vi "CmdExe.Launch Executable with Timeout, Abort, and Error Checks - Using DotNet Process.vi"(5 "Cmd IN Ref":refnum<vi>, 6 "Setup":T1={"Timeout (s)"=60.0, "Show Cmd Win"=FALSE, "Error Check"={"StdOut_Ck"=FALSE, "StdOutErrMsgs"=["Error", "Unable to find device "], "StdErr_Ck"=FALSE, "RtnCode_Ck"=FALSE, "RtnCodePASS"=0}, "Log_En"=FALSE, "LogFileName"="", "LogDir"=path ""}, 7 "Output Ref":refnum<vi>, 8 "error in (no error)":errorcluster, 9 "Ignore StdErr":bool, 10 "Args":string="/InputFile JSONFILE /SerialDevice /OutputDevice /NoBackup", 11 "Executable":path=path "C:/MTE/FW Load and Display Cal/Config/Bin/utahev_0_7/lighthouse_configtool.exe") -> (0 "error out":errorcluster, 1 "Duration(s)":dbl, 3 "Data Out":string)   [LabVIEW 2018]
uses:
  <vilib>/KATE/Time/Time Utils.lvlib
  Errors/Error.Error Code List.ctl
  <vilib>/KATE/Files/File Utils.lvlib
  CmdConsole/CmdConsole.lvclass
  CmdExe.Setup Params.ctl
  CmdExe.Output Error Check Setup.ctl
panel:
  out "return code":i32
  out "Cmd":string
  out "Done":bool
  # "Launch Exe"
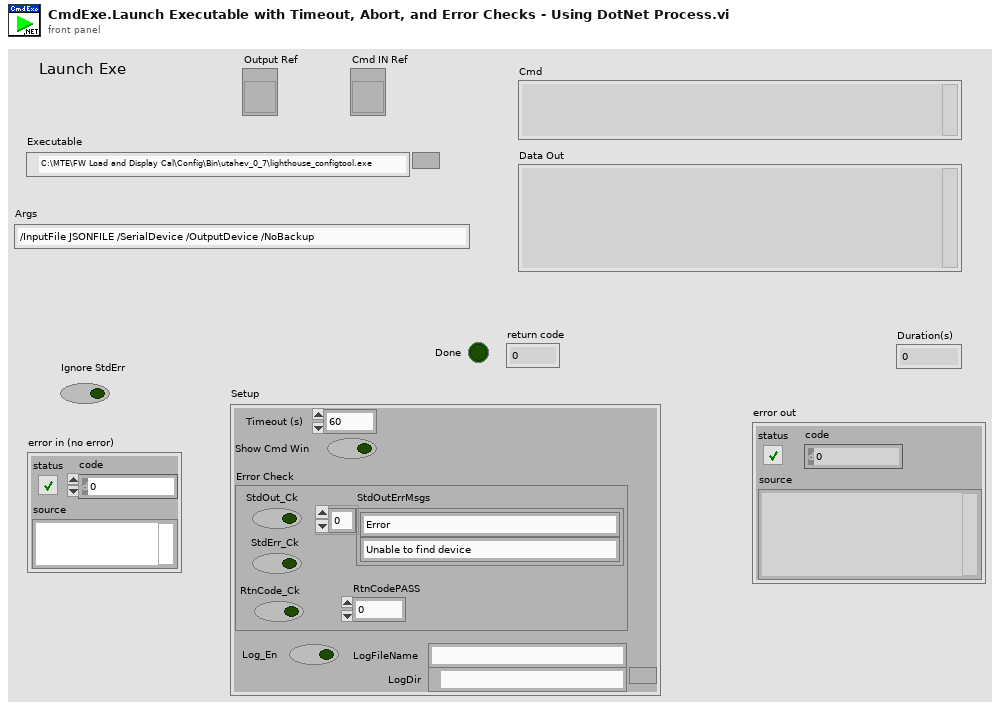
[diagram p1: front panel]
types:
  T1 = typedef "CmdExe.Setup Params.ctl" = cluster{"Timeout (s)":dbl, "Show Cmd Win":bool, "Error Check":T2, "Log_En":bool, "LogFileName":string, "LogDir":path}
  T2 = typedef "CmdExe.Output Error Check Setup.ctl" = cluster{"StdOut_Ck":bool, "StdOutErrMsgs":string[], "StdErr_Ck":bool, "RtnCode_Ck":bool, "RtnCodePASS":i32}
  T3 = enum16{"open", "replace", "create", "open or create", "replace or create", "replace or create with confirmation"}
  T4 = cluster{"Exe":string, "StdOut":string, "StdError":string, "LogFile":path, "Args":string, "TimedOut":bool, "RtnCode":i32, "LogEn":bool}
  T5 = typedef "Error.Error Code List.ctl" = i32
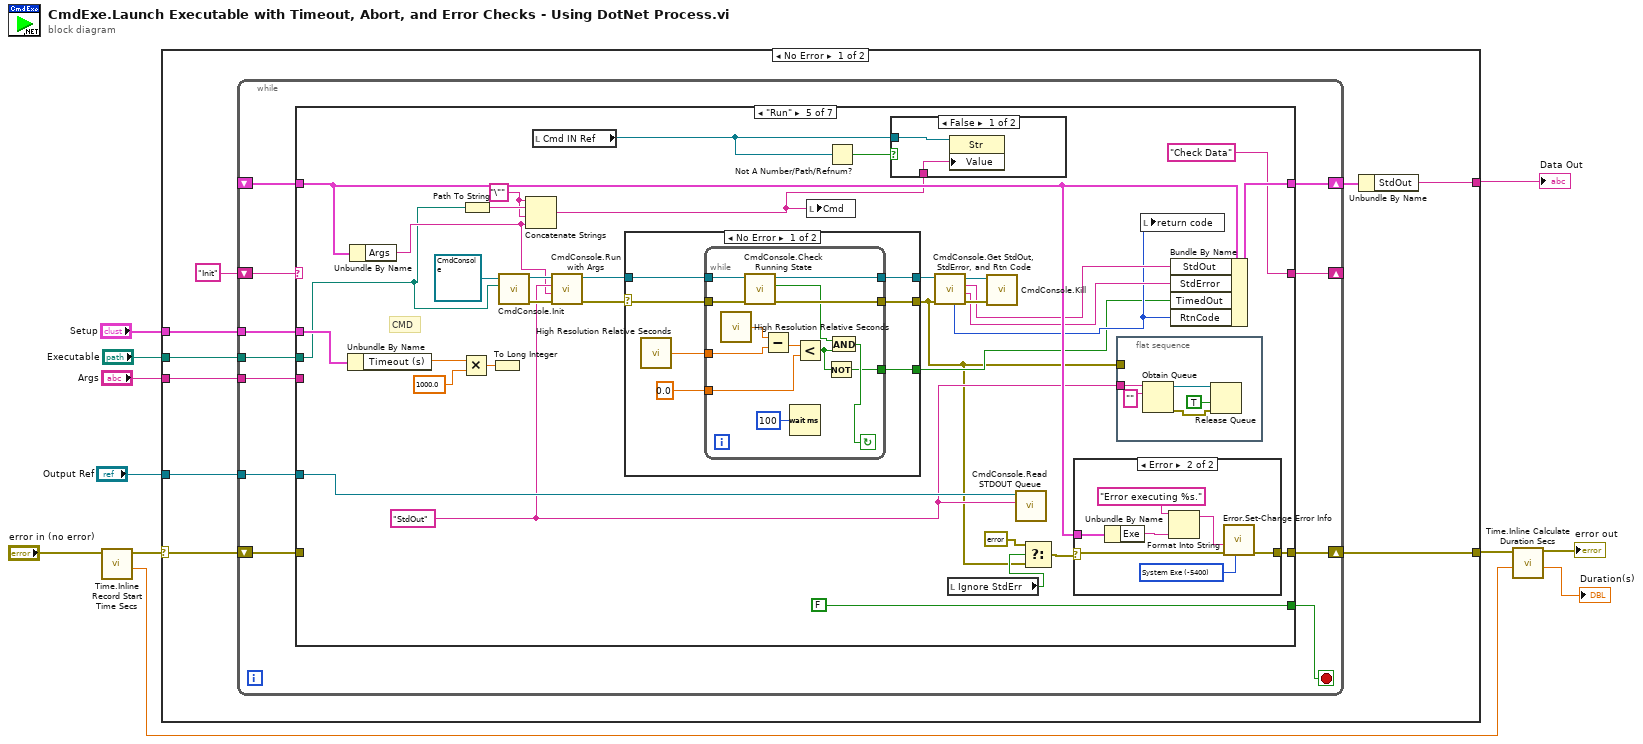
[diagram p0: block diagram]
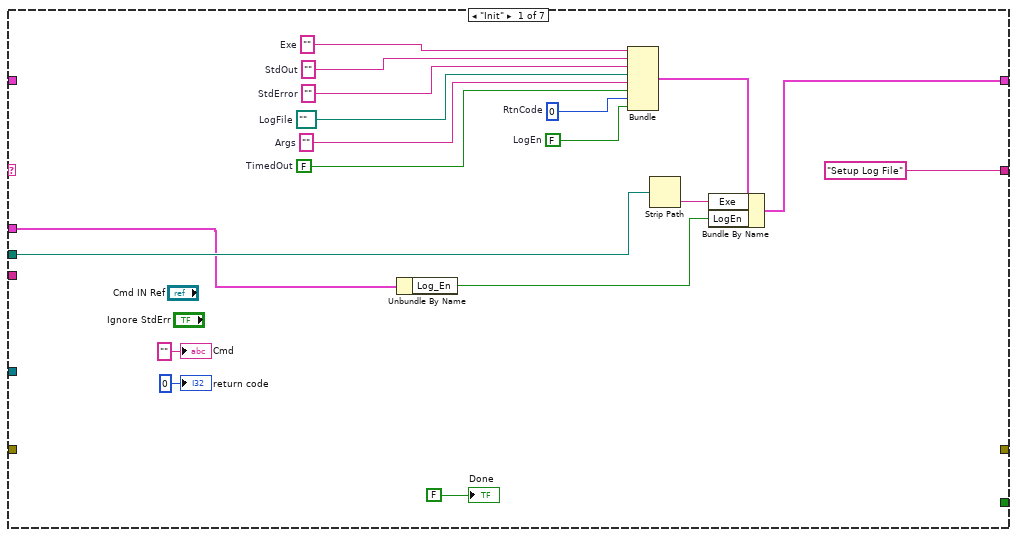
[diagram p2: hidden frame]
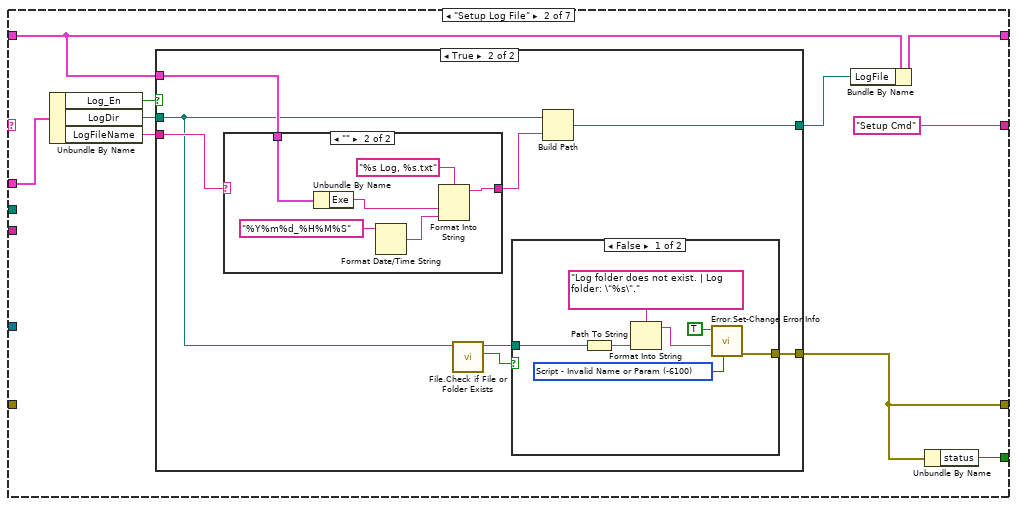
[diagram p3: hidden frame]
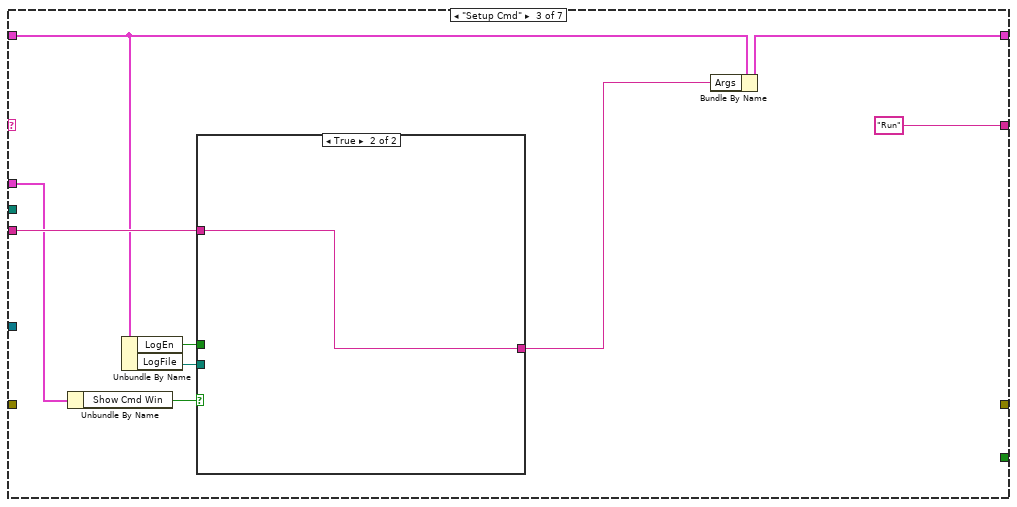
[diagram p7: hidden frame]
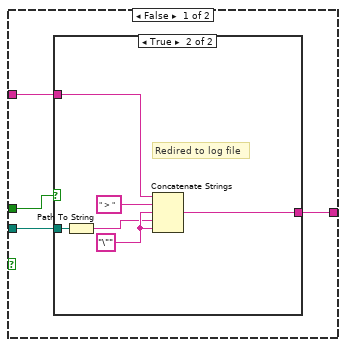
[diagram p8: hidden frame]
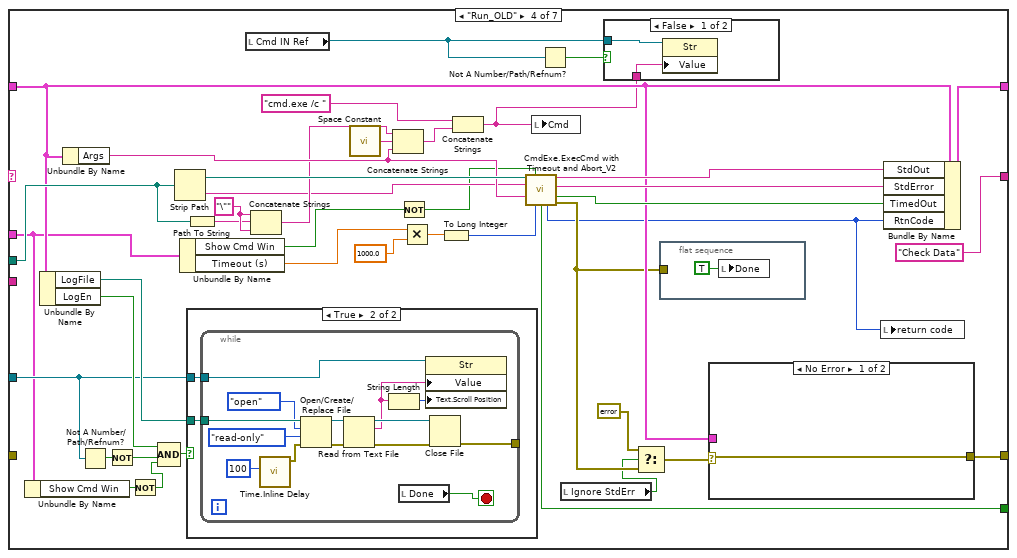
[diagram p10: hidden frame]
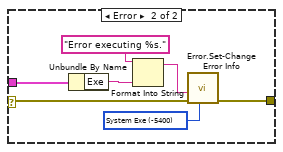
[diagram p11: hidden frame]
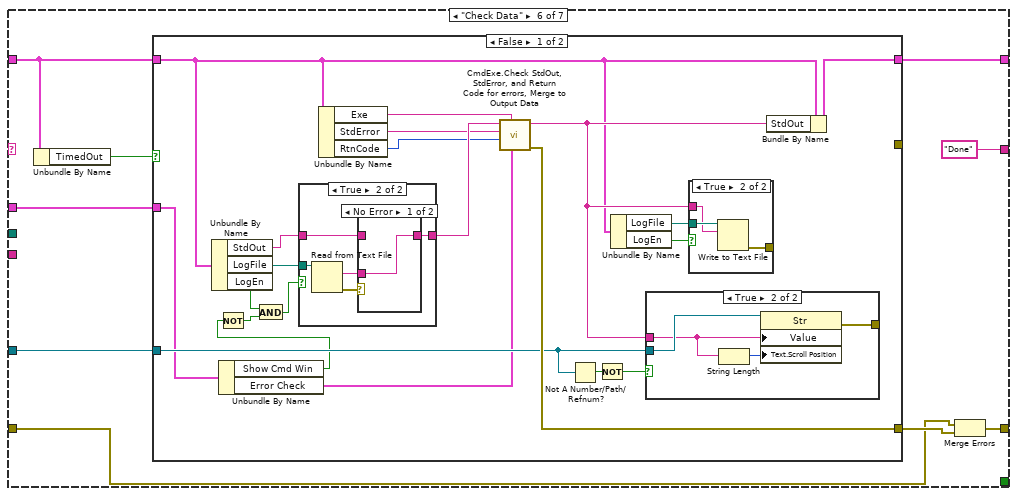
[diagram p17: hidden frame]
diagram:
  n1 = call <vilib>:"Time.Inline Record Start Time Secs.vi"("Error In Upper"="error in (no error)") -> ("Start(s)"=w8:dbl, "Error Out Upper"=w11:errorcluster)  [unwired: 8 in, 1 out]
  n2 = case shown="No Error" w11 {
    selector: w11 -> [w19 w318]
    tunnel: [w18 w318] -> w10
    tunnel: [w16 _] -> w9
    tunnel: "Executable" -> [w15 _]
    tunnel: "Args" -> [w14 _]
    tunnel: "Setup" -> [w13 _]
    tunnel: "Output Ref" -> [w12 _]
    frame No Error {
      n3 = while {
        shift-right: [w29] -> w17
        shift-left: _ -> [w28]
        shift-right: [w21] -> _
        shift-left: "Init" -> [w31]
        shift-right: [w27] -> w18
        shift-left: w19 -> [w30]
        tunnel: w15 -> [w25]
        tunnel: w14 -> [w24]
        tunnel: w13 -> [w23]
        tunnel: w12 -> [w22]
        stop <- w26 stop-if-true
        n4 = case shown="\"Run\"" w31 {
          tunnel: ["Setup Log File" "Setup Cmd" "Run" "Check Data" "Check Data" "Done" "Done"] -> w21
          tunnel: w30 -> [_ _ _ _ _ w242 w314]
          tunnel: [w38 w58 w89 w143 w204 w250 w315] -> w29
          tunnel: [_ w51 _ w114 w196 w244 w314] -> w27
          tunnel: w28 -> [_ w56 w84 w113 w195 w248 w315]
          tunnel: [_ w50 _ w139 FALSE _ TRUE] -> w26
          tunnel: w25 -> [w41 _ _ w127 w177 _ _]
          tunnel: w24 -> [_ _ w87 _ _ _ _]
          tunnel: w23 -> [w35 w55 w83 w109 w192 w246 _]
          tunnel: w22 -> [_ _ _ w115 w197 w249 _]
          frame "Init" {
            w36 = FALSE  # LogEn
            w37 = 0  # RtnCode
            w42 = FALSE  # TimedOut
            w43 = ""  # Args
            w44 = path ""  # LogFile
            w45 = ""  # StdError
            w46 = ""  # StdOut
            w48 = ""  # Exe
            n5 = Unbundle By Name(w35) -> ("Log_En"=w34:bool)
            n6 = Bundle("Exe"=w48, "StdOut"=w46, "StdError"=w45, "LogFile"=w44, "Args"=w43, "TimedOut"=w42, "RtnCode"=w37, "LogEn"=w36) -> (w39:T4)  [unwired: 1 in]
            n7 = Strip Path(path=w41) -> (name=w40:string)  [unwired: 1 out]
            n8 = Bundle By Name(cluster=w39, "Exe"=w40, "LogEn"=w34) -> (w38:T4)
            "Done" <- FALSE ("Done")
            "Cmd" <- "" ("Cmd")
            "return code" <- 0 ("return code")
          }
          frame "Setup Log File" {
            n9 = Unbundle By Name(w55) -> ("Log_En"=w54:bool, "LogDir"=w53:path, "LogFileName"=w52:string)
            n10 = case shown="True" w54 {
              tunnel: [_ w67] -> w57
              tunnel: w56 -> [_ w65]
              tunnel: w53 -> [_ w61]
              tunnel: w52 -> [_ w64]
              tunnel: [_ w60] -> w51
              frame False {
              }
              frame True {
                n11 = case shown="\"\"" w64 {
                  selector: w64 -> [w75 _]
                  tunnel: [w75 w78] -> w66
                  tunnel: w65 -> [_ w77]
                  frame Default {
                  }
                  frame "" {
                    n12 = Unbundle By Name(w77) -> ("Exe"=w76:string)
                    n13 = Format Date/Time String(time format string (%c)="%Y%m%d_%H%M%S") -> (date/time string=w81:string)  [unwired: 2 in]
                    n14 = Format Into String(format string="%s Log, %s.txt", w76, w81) -> (resulting string=w78:string)  [unwired: 2 in, 1 out]
                  }
                }
                n15 = call <vilib>:"File.Check if File or Folder Exists.vi"("Path"=w61) -> ("Exists"=w62:bool, "Dup Path"=w63:path)  [unwired: 6 in, 3 out]
                n16 = case shown="False" w62 {
                  tunnel: [w68 _] -> w60
                  tunnel: w63 -> [w72 _]
                  frame False {
                    w70 = T5 -6100 items=["No Error"=0, "Abort"=-2, "Misc"=-5000, "Fixture Error"=-5100, "File IO - General"=-5200, "FIle IO - Config Error"=-5201, "Instrument - General"=-5300, "Instrument - Serial Com"=-5301, "Instrument - Camera"=-5302, "Instrument - PS"=-5303, "Instrument - Oscilloscope"=-5304, "Instrument - Function Gen"=-5305, "Instrument - Load"=-5306, "Instrument - Meter"=-5307, "Instrument - Power Control"=-5308, "Instrument - Motion"=-5309, "Instrument - RF"=-5310, "System Exe"=-5400, "Image Processing"=-5500, "Communication"=-5600, "Script - Syntax Error"=-6000, "Script - Invalid Name or Param"=-6100, "Script - Timeout"=-6200, "Invalid Data"=-6300] ("Std Code")
                    n17 = Path To String(path=w72) -> (string=w73:string)
                    n18 = Format Into String(format string="Log folder does not exist. | Log folder: \"%s\".", w73) -> (resulting string=w69:string)  [unwired: 2 in, 1 out]
                    n19 = call "Error.Set-Change Error Info.vi"("Std Code"=w70, "Description"=w69, "Set Error"=TRUE) -> ("error out"=w68:errorcluster)  [unwired: 8 in]
                  }
                  frame True {
                    # "Folders exist.\nNo error."
                  }
                }
                n20 = Build Path(base path=w61, name or relative path=w66) -> (appended path=w67:path)
              }
            }
            n21 = Bundle By Name(cluster=w56, "LogFile"=w57) -> (w58:T4)
            n22 = Unbundle By Name(w51) -> ("status"=w50:bool)
          }
          frame "Setup Cmd" {
            n23 = Unbundle By Name(w83) -> ("Show Cmd Win"=w82:bool)
            n24 = Unbundle By Name(w84) -> ("LogEn"=w85:bool, "LogFile"=w88:path)
            n25 = case shown="True" w82 {
              tunnel: w88 -> [w94 _]
              tunnel: w87 -> [w93 w102]
              tunnel: [w92 w102] -> w86
              tunnel: w85 -> [w91 _]
              frame False {
                n26 = case shown="True" w91 {
                  tunnel: w94 -> [_ w98]
                  tunnel: w93 -> [w95 w97]
                  tunnel: [w95 w96] -> w92
                  frame False {
                  }
                  frame True {
                    w101 = "\""
                    # "Redired to log file"
                    n27 = Path To String(path=w98) -> (string=w100:string)
                    n28 = Concatenate Strings(w97, " > ", w101, w100, w101) -> (w96:string)
                  }
                }
              }
              frame True {
              }
            }
            n29 = Bundle By Name(cluster=w84, "Args"=w86) -> (w89:T4)
          }
          frame "Run_OLD" {
            w128 = "\""
            n30 = Unbundle By Name(w109) -> ("Show Cmd Win"=w108:bool)
            n31 = Unbundle By Name(w113) -> ("LogFile"=w134:path, "LogEn"=w120:bool)
            n32 = Unbundle By Name(w113) -> ("Args"=w129:string)
            n33 = Not A Number/Path/Refnum?(number/path/refnum=w115) -> (NaN/Path/Refnum?=w123:bool)
            n34 = Not(x=w123) -> (.not. x?=w122:bool)
            n35 = Not(x=w108) -> (.not. x?=w107:bool)
            n36 = Compound Arithmetic op=AND(w120, w122, w107) -> (w121:bool)
            n37 = Strip Path(path=w127) -> (stripped path=w133:path, name=w124:string)
            n38 = Unbundle By Name(w109) -> ("Show Cmd Win"=w118:bool, "Timeout (s)"=w119:dbl)
            n39 = Path To String(path=w127) -> (string=w126:string)
            n40 = case shown="True" w121 {
              tunnel: w134 -> [_ w155]
              tunnel: w115 -> [_ w156]
              frame False {
              }
              frame True {
                n41 = while {
                  tunnel: w156 -> [w162]
                  tunnel: w155 -> [w166]
                  tunnel: [w165] -> _
                  stop <- w161 stop-if-true
                  n42 = call <vilib>:"Time.Inline Delay.vi"("Wait(ms)"=u32 100) -> ("error out top"=w159:errorcluster)  [unwired: 9 in, 1 out]
                  n43 = Open/Create/Replace File(file path (use dialog)=w166, error in=w159, operation (0:open)=T3."open", access (0:read/write)=enum16{"read/write", "read-only", "write-only"}."read-only") -> (refnum out=w167:refnum<file>, error out=w170:errorcluster)  [unwired: 2 in, 1 out]
                  n44 = Read from Text File(file (use dialog)=w167, error in=w170) -> (refnum out=w168:refnum<file>, text=w158:string, error out=w169:errorcluster)  [unwired: 2 in, 1 out]
                  n45 = String Length(string=w158) -> (length=w157:i32)
                  n46 = local read "Done"() -> (w161:bool)
                  n47 = property class="Str"(reference=w162, "Value"=w158, "Text.Scroll Position"=w157) -> ()  [unwired: 1 in, 2 out]
                  n48 = Close File(refnum=w168, error in=w169) -> (error out=w165:errorcluster)  [unwired: 1 out]
                }
              }
            }
            n49 = local read "Cmd IN Ref"() -> (w106:refnum<vi>)
            n50 = Concatenate Strings(w128, w126, w128) -> (w125:string)
            n51 = call <vilib>:"Space Constant.vi"() -> ("String"=w130:string)
            n52 = Concatenate Strings(w125, w130, w129) -> (w131:string)
            n53 = Not(x=w118) -> (.not. x?=w117:bool)
            n54 = Multiply(x=w119, y=1000.0) -> (x*y=w138:dbl)
            n55 = To Long Integer(number=w138) -> (32bit integer=w136:i32)
            n56 = Concatenate Strings("cmd.exe /c ", w131) -> (w103:string)
            n57 = call "CmdExe.ExecCmd with Timeout and Abort_V2.vi"("Working Dir"=w133, "Run minimized? (T)"=w117, "Executable"=w124, "Arguements"=w129, "Timeout ms(-1)"=w136) -> ("STD OUT"=w116:string, "STD ERR"=w142:string, "Timed Out"=w141:bool, "Aborted"=w139:bool, "return code"=w104:i32, "error out"=w112:errorcluster)  [unwired: 5 in]
            n58 = local write "Cmd"(w103) -> ()
            n59 = Not A Number/Path/Refnum?(number/path/refnum=w106) -> (NaN/Path/Refnum?=w135:bool)
            n60 = local read "Ignore StdErr"() -> (w105:bool)
            n61 = case shown="False" w135 {
              tunnel: w106 -> [w154 _]
              tunnel: w103 -> [w153 _]
              frame False {
                n62 = property class="Str"(reference=w154, "Value"=w153) -> ()  [unwired: 1 in, 2 out]
              }
              frame True {
              }
            }
            n63 = Select(t=errorcluster {"status"=FALSE, "code"=0, "source"=""}, s=w105, f=w112) -> (s? t:f=w111:errorcluster)
            n64 = flat-sequence {
              tunnel: w112 -> [_]
              frame #0 {
                n65 = local write "Done"(TRUE ("Done")) -> ()
              }
            }
            n66 = case shown="No Error" w111 {
              selector: w111 -> [w144 w147]
              tunnel: [w144 w146] -> w114
              tunnel: w113 -> [_ w145]
              frame No Error {
              }
              frame Error {
                w149 = T5 -5400 items=["No Error"=0, "Abort"=-2, "Misc"=-5000, "Fixture Error"=-5100, "File IO - General"=-5200, "FIle IO - Config Error"=-5201, "Instrument - General"=-5300, "Instrument - Serial Com"=-5301, "Instrument - Camera"=-5302, "Instrument - PS"=-5303, "Instrument - Oscilloscope"=-5304, "Instrument - Function Gen"=-5305, "Instrument - Load"=-5306, "Instrument - Meter"=-5307, "Instrument - Power Control"=-5308, "Instrument - Motion"=-5309, "Instrument - RF"=-5310, "System Exe"=-5400, "Image Processing"=-5500, "Communication"=-5600, "Script - Syntax Error"=-6000, "Script - Invalid Name or Param"=-6100, "Script - Timeout"=-6200, "Invalid Data"=-6300] ("Std Code")
                n67 = Unbundle By Name(w145) -> ("Exe"=w150:string)
                n68 = Format Into String(format string="Error executing %s.", w150) -> (resulting string=w148:string)  [unwired: 2 in, 1 out]
                n69 = call "Error.Set-Change Error Info.vi"("Std Code"=w149, "error in"=w147, "Description"=w148) -> ("error out"=w146:errorcluster)  [unwired: 8 in]
              }
            }
            n70 = local write "return code"(w104) -> ()
            n71 = Bundle By Name(cluster=w113, "StdOut"=w116, "StdError"=w142, "TimedOut"=w141, "RtnCode"=w104) -> (w143:T4)
          }
          frame "Run" {
            w179 = "StdOut" ("QName")
            w188 = "\""
            # "CMD"
            n72 = Unbundle By Name(w192) -> ("Timeout (s)"=w198:dbl)
            n73 = Unbundle By Name(w195) -> ("Args"=w178:string)
            n74 = Multiply(x=w198, y=1000.0) -> (x*y=w202:dbl)
            n75 = Path To String(path=w177) -> (string=w199:string)
            n76 = To Long Integer(number=w202) -> ()  [unwired: 1 out]
            n77 = call "CmdConsole.Init.vi"("App"=w177, "CmdConsole in"=refnum<class "CmdConsole.lvclass"> refnum) -> ("error out"=w182:errorcluster, "CmdConsole out"=w181:refnum<class "CmdConsole.lvclass">)  [unwired: 8 in]
            n78 = Concatenate Strings(w188, w199, w188, w178) -> (w189:string)
            n79 = local read "Cmd IN Ref"() -> (w191:refnum<vi>)
            n80 = call "CmdConsole.Run with Args.vi"("error in (no error)"=w182, "Args"=w178, "StdOutQ"=w179, "CmdConsole in"=w181) -> ("error out"=w184:errorcluster, "CmdConsole out"=w183:refnum<class "CmdConsole.lvclass">)  [unwired: 5 in, 1 out]
            n81 = case shown="No Error" w184 {
              selector: w184 -> [w206 w225]
              tunnel: w183 -> [w211 w226]
              tunnel: [w210 w225] -> w172
              tunnel: [w209 w226] -> w185
              tunnel: [w205 _] -> w173
              frame No Error {
                n82 = call <vilib>:"High Resolution Relative Seconds.vi"() -> ("relative seconds"=w208:dbl)
                n83 = while {
                  tunnel: w211 -> [w224]
                  tunnel: w206 -> [w223]
                  tunnel: [w222] -> w210
                  tunnel: [w221] -> w209
                  tunnel: w208 -> [w219]
                  tunnel: 0.0 -> [w217]
                  tunnel: [w212] -> w205
                  stop <- w215 continue-if-true
                  n84 = call <vilib>:"High Resolution Relative Seconds.vi"() -> ("relative seconds"=w220:dbl)
                  n85 = call "CmdConsole.Check Running State.vi"("error in (no error)"=w223, "CmdConsole in"=w224) -> ("error out"=w222:errorcluster, "Running"=w216:bool, "CmdConsole out"=w221:refnum<class "CmdConsole.lvclass">)  [unwired: 7 in]
                  n86 = Subtract(x=w220, y=w219) -> (x-y=w218:dbl)
                  n87 = Wait (ms)(milliseconds to wait=u32 100) -> ()  [unwired: 1 out]
                  n88 = Less?(x=w218, y=w217) -> (x < y?=w213:bool)
                  n89 = Not(x=w213) -> (.not. x?=w212:bool)
                  n90 = And(x=w216, y=w213) -> (x .and. y?=w215:bool)
                }
              }
              frame Error {
              }
            }
            n91 = local write "Cmd"(w189) -> ()
            n92 = Not A Number/Path/Refnum?(number/path/refnum=w191) -> (NaN/Path/Refnum?=w200:bool)
            n93 = case shown="False" w200 {
              tunnel: w191 -> [w241 _]
              tunnel: w189 -> [w240 _]
              frame False {
                n94 = property class="Str"(reference=w241, "Value"=w240) -> ()  [unwired: 1 in, 2 out]
              }
              frame True {
              }
            }
            n95 = call "CmdConsole.Get StdOut, StdError, and Rtn Code.vi"("error in (no error)"=w172, "CmdConsole in"=w185) -> ("error out"=w186:errorcluster, "StdErr"=w175:string, "StdOut"=w176:string, "CmdConsole out"=w187:refnum<class "CmdConsole.lvclass">, "Rtn Code"=w174:i32)  [unwired: 5 in]
            n96 = local read "Ignore StdErr"() -> (w190:bool)
            n97 = call "CmdConsole.Kill.vi"("error in"=w186, "CmdConsole in"=w187) -> ()  [unwired: 8 in, 2 out]
            n98 = call "CmdConsole.Read STDOUT Queue.vi"("QName"=w179, "StdOut Ctrl"=w197) -> ()  [unwired: 10 in]
            n99 = Select(t=errorcluster {"status"=FALSE, "code"=0, "source"=""}, s=w190, f=w172) -> (s? t:f=w194:errorcluster)
            n100 = case shown="Error" w194 {
              selector: w194 -> [w227 w230]
              tunnel: [w227 w229] -> w196
              tunnel: w195 -> [_ w228]
              frame No Error {
              }
              frame Error {
                w232 = T5 -5400 items=["No Error"=0, "Abort"=-2, "Misc"=-5000, "Fixture Error"=-5100, "File IO - General"=-5200, "FIle IO - Config Error"=-5201, "Instrument - General"=-5300, "Instrument - Serial Com"=-5301, "Instrument - Camera"=-5302, "Instrument - PS"=-5303, "Instrument - Oscilloscope"=-5304, "Instrument - Function Gen"=-5305, "Instrument - Load"=-5306, "Instrument - Meter"=-5307, "Instrument - Power Control"=-5308, "Instrument - Motion"=-5309, "Instrument - RF"=-5310, "System Exe"=-5400, "Image Processing"=-5500, "Communication"=-5600, "Script - Syntax Error"=-6000, "Script - Invalid Name or Param"=-6100, "Script - Timeout"=-6200, "Invalid Data"=-6300] ("Std Code")
                n101 = Unbundle By Name(w228) -> ("Exe"=w233:string)
                n102 = Format Into String(format string="Error executing %s.", w233) -> (resulting string=w231:string)  [unwired: 2 in, 1 out]
                n103 = call "Error.Set-Change Error Info.vi"("Std Code"=w232, "error in"=w230, "Description"=w231) -> ("error out"=w229:errorcluster)  [unwired: 8 in]
              }
            }
            n104 = flat-sequence {
              tunnel: w172 -> [_]
              tunnel: w179 -> [w236]
              frame #0 {
                n105 = Obtain Queue(name (unnamed)=w236, element data type="") -> (queue out=w239:refnum<queue>, error out=w237:errorcluster)  [unwired: 3 in, 1 out]
                n106 = Release Queue(queue=w239, force destroy? (F)=TRUE, error in (no error)=w237) -> ()  [unwired: 3 out]
              }
            }
            n107 = local write "return code"(w174) -> ()
            n108 = Bundle By Name(cluster=w195, "StdOut"=w176, "StdError"=w175, "TimedOut"=w173, "RtnCode"=w174) -> (w204:T4)
          }
          frame "Check Data" {
            n109 = Unbundle By Name(w248) -> ("TimedOut"=w247:bool)
            n110 = case shown="False" w247 {
              tunnel: [w271 w293] -> w250
              tunnel: w248 -> [w255 w287]
              tunnel: [w266 w298] -> w243
              tunnel: w249 -> [w263 _]
              tunnel: w246 -> [w260 w303]
              tunnel: [_ w288] -> _
              frame False {
                n111 = Unbundle By Name(w255) -> ("StdOut"=w261:string, "LogFile"=w270:path, "LogEn"=w254:bool)
                n112 = Unbundle By Name(w260) -> ("Show Cmd Win"=w252:bool, "Error Check"=w259:T2)
                n113 = Not(x=w252) -> (.not. x?=w253:bool)
                n114 = And(x=w254, y=w253) -> (x .and. y?=w251:bool)
                n115 = case shown="True" w251 {
                  tunnel: w270 -> [_ w284]
                  tunnel: [w279 w282] -> w269
                  tunnel: w261 -> [w279 w280]
                  frame False {
                    (unwired) TRUE
                  }
                  frame True {
                    n116 = Read from Text File(file (use dialog)=w284) -> (text=w281:string, error out=w283:errorcluster)  [unwired: 3 in, 2 out]
                    n117 = case shown="No Error" w283 {
                      tunnel: [w285 w286] -> w282
                      tunnel: w281 -> [w285 _]
                      tunnel: w280 -> [_ w286]
                      frame No Error {
                      }
                      frame Error {
                      }
                    }
                  }
                }
                n118 = Unbundle By Name(w255) -> ("Exe"=w262:string, "StdError"=w268:string, "RtnCode"=w267:i32)
                n119 = call "CmdExe.Check StdOut, StdError, and Return Code for errors, Merge to Output Data.vi"("Error Check"=w259, "App Name"=w262, "Return Code"=w267, "StdError"=w268, "StdOut"=w269) -> ("error out"=w266:errorcluster, "Output Data"=w256:string)  [unwired: 5 in]
                n120 = Not A Number/Path/Refnum?(number/path/refnum=w263) -> (NaN/Path/Refnum?=w265:bool)
                n121 = Not(x=w265) -> (.not. x?=w264:bool)
                n122 = Unbundle By Name(w255) -> ("LogFile"=w258:path, "LogEn"=w257:bool)
                n123 = case shown="True" w264 {
                  tunnel: w263 -> [_ w277]
                  tunnel: w256 -> [_ w276]
                  tunnel: [_ w275] -> _
                  frame False {
                  }
                  frame True {
                    n124 = String Length(string=w276) -> (length=w278:i32)
                    n125 = property class="Str"(reference=w277, "Value"=w276, "Text.Scroll Position"=w278) -> (error out=w275:errorcluster)  [unwired: 1 in, 1 out]
                  }
                }
                n126 = case shown="True" w257 {
                  tunnel: w258 -> [_ w274]
                  tunnel: [_ w273] -> _
                  tunnel: w256 -> [_ w272]
                  frame False {
                    (unwired) TRUE
                  }
                  frame True {
                    n127 = Write to Text File(file (use dialog)=w274, text=w272) -> (error out=w273:errorcluster)  [unwired: 2 in, 2 out]
                  }
                }
                n128 = Bundle By Name(cluster=w255, "StdOut"=w256) -> (w271:T4)
              }
              frame True {
                w301 = T5 -5400 items=["No Error"=0, "Abort"=-2, "Misc"=-5000, "Fixture Error"=-5100, "File IO - General"=-5200, "FIle IO - Config Error"=-5201, "Instrument - General"=-5300, "Instrument - Serial Com"=-5301, "Instrument - Camera"=-5302, "Instrument - PS"=-5303, "Instrument - Oscilloscope"=-5304, "Instrument - Function Gen"=-5305, "Instrument - Load"=-5306, "Instrument - Meter"=-5307, "Instrument - Power Control"=-5308, "Instrument - Motion"=-5309, "Instrument - RF"=-5310, "System Exe"=-5400, "Image Processing"=-5500, "Communication"=-5600, "Script - Syntax Error"=-6000, "Script - Invalid Name or Param"=-6100, "Script - Timeout"=-6200, "Invalid Data"=-6300] ("Std Code")
                n129 = Unbundle By Name(w303) -> ("Timeout (s)"=w302:dbl)
                n130 = Unbundle By Name(w287) -> ("StdOut"=w290:string, "LogFile"=w292:path, "LogEn"=w291:bool)
                n131 = Unbundle By Name(w287) -> ("Exe"=w304:string)
                n132 = Unbundle By Name(w287) -> ("Exe"=w295:string, "StdError"=w297:string, "RtnCode"=w296:i32)
                n133 = case shown="True" w291 {
                  tunnel: w292 -> [_ w311]
                  tunnel: [w306 w309] -> w289
                  tunnel: w290 -> [w306 w307]
                  frame False {
                    (unwired) TRUE
                  }
                  frame True {
                    n134 = Read from Text File(file (use dialog)=w311) -> (text=w308:string, error out=w310:errorcluster)  [unwired: 3 in, 2 out]
                    n135 = case shown="No Error" w310 {
                      tunnel: [w312 w313] -> w309
                      tunnel: w308 -> [w312 _]
                      tunnel: w307 -> [_ w313]
                      frame No Error {
                      }
                      frame Error {
                      }
                    }
                  }
                }
                n136 = Format Into String(format string="%s was terminated due to timeout (%.1f secs).  ", w304, w302) -> (resulting string=w299:string)  [unwired: 2 in, 1 out]
                n137 = call "CmdExe.Check StdOut, StdError, and Return Code for errors, Merge to Output Data.vi"("App Name"=w295, "Return Code"=w296, "StdError"=w297, "StdOut"=w289) -> ("error out"=w288:errorcluster, "Output Data"=w294:string)  [unwired: 6 in]
                n138 = call "Error.Set-Change Error Info.vi"("Std Code"=w301, "Description"=w299, "Set Error"=TRUE) -> ("error out"=w298:errorcluster)  [unwired: 8 in]
                n139 = Bundle By Name(cluster=w287, "StdOut"=w294) -> (w293:T4)
              }
            }
            n140 = Merge Errors(w242, w243) -> (w244:errorcluster)
          }
          frame "Done", Default {
          }
        }
      }
      n141 = Unbundle By Name(w17) -> ("StdOut"=w16:string)
    }
    frame Error {
    }
  }
  "Data Out" <- w9
  n142 = call <vilib>:"Time.Inline Calculate Duration Secs.vi"("Start(Sec)"=w8, "Error In Top"=w10) -> ("Duration(s)"=→"Duration(s)":dbl, "Error Out Top"=→"error out":errorcluster)  [unwired: 7 in, 1 out]
